vi "Get Config.vi"(8 "error in (no error)":errorcluster, 11 "VisaResource in":refnum<class "VisaResource.lvclass">) -> (0 "error out":errorcluster, 2 "Config":T1[](array[typedef]), 3 "VisaResource out":refnum<class "VisaResource.lvclass">)   [LabVIEW 2020, in "PicoG-Core.lvlib" / "VisaResource.lvclass"]
uses:
  VisaResource.lvclass
  Resource/Config Item.ctl
  VisaResource.lvclass/VisaResource.ctl
  Resource/Resource.lvclass
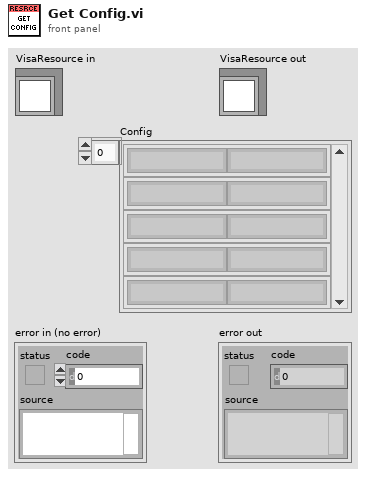
[diagram p1: front panel]
types:
  T1 = typedef "PicoG-Core.lvlib/Resource.lvclass/Config Item.ctl" = cluster{"Key":string, "Value":string}
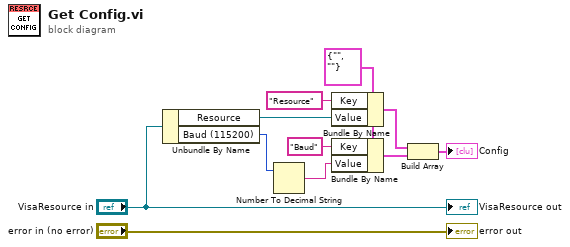
[diagram p0: block diagram]
diagram:
  w8 = T1 {"Key"="", "Value"=""} ("Config Item")
  n1 = Unbundle By Name("VisaResource in") -> ("Resource"=w7:refnum<visa-resource-name>, "Baud (115200)"=w9:u32)
  n2 = Number To Decimal String(number=w9) -> (decimal integer string=w4:string)  [unwired: 1 in]
  n3 = Bundle By Name(cluster=w8, "Key"="Resource", "Value"=w7) -> (w3:T1)
  n4 = Bundle By Name(cluster=w8, "Key"="Baud", "Value"=w4) -> (w2:T1)
  n5 = Build Array(w3, w2) -> (→"Config":T1[])
  "error out" <- "error in (no error)"
  "VisaResource out" <- "VisaResource in"
